vi "Get Displacement Profile.vi"(8 "R2":dbl, 9 "R12":dbl, 10 "r":dbl[](array[numeric]), 11 "xd'":dbl) -> (3 "xd (r)":dbl[](array[numeric]))   [LabVIEW 2022 SP3]
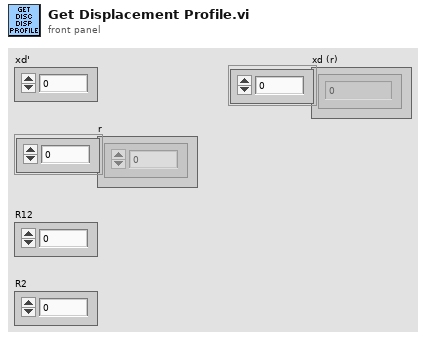
[diagram p1: front panel]
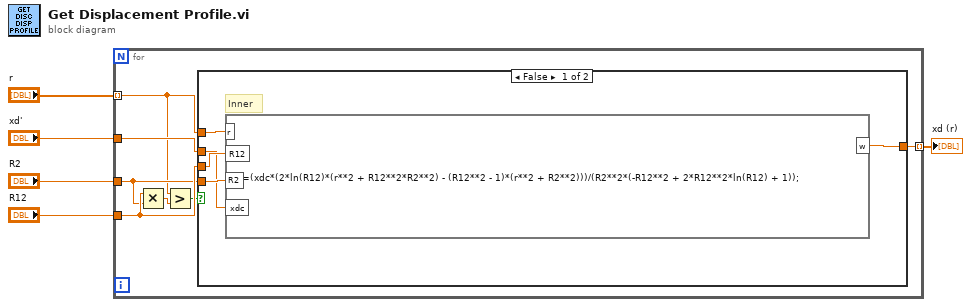
[diagram p0: block diagram]
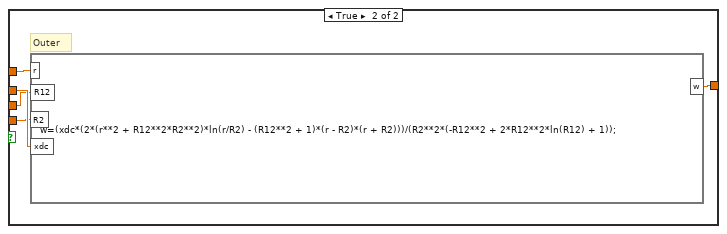
[diagram p2: hidden frame]
diagram:
  n1 = for {
    tunnel: "r" -> [w8] mode=indexing
    tunnel: "xd'" -> [w12]
    tunnel: "R2" -> [w10]
    tunnel: "R12" -> [w11]
    tunnel: [w6] -> w4 mode=indexing
    n2 = Multiply(x=w11, y=w10) -> (x*y=w9:dbl)
    n3 = Greater?(x=w8, y=w9) -> (0:w7:bool)
    n4 = case shown="False" w7 {
      tunnel: w12 -> [w14 w22]
      tunnel: w11 -> [w16 w21]
      tunnel: w10 -> [w15 w20]
      tunnel: w8 -> [w17 w19]
      tunnel: [w13 w18] -> w6
      frame False {
        # "Inner"
        n5 = formula code="w=(xdc*(2*ln(R12)*(r**2 + R12**2*R2**2) - (R12**2 - 1)*(r**2 + R2**2)))/(R2**2*(-R12**2 + 2*R12**2*ln(R12) + 1));"("r"=w17, "R12"=w16, "R2"=w15, "xdc"=w14) -> ("w"=w13:dbl)
      }
      frame True {
        # "Outer"
        n6 = formula code="w=(xdc*(2*(r**2 + R12**2*R2**2)*ln(r/R2) - (R12**2 + 1)*(r - R2)*(r + R2)))/(R2**2*(-R12**2 + 2*R12**2*ln(R12) + 1));"("r"=w19, "R12"=w21, "R2"=w20, "xdc"=w22) -> ("w"=w18:dbl)
      }
    }
  }
  "xd (r)" <- w4
